vi "Run Tests (Path).vi"(8 "error in (no error)":errorcluster, 10 "Project or Class Path":path, 11 "Execution API In":refnum<class "Execution API.lvclass">) -> (0 "error out":errorcluster, 3 "Execution API Out":refnum<class "Execution API.lvclass">)   [LabVIEW 2020, in "Execution API.lvclass"]
doc: "Run all tests in a project or a test case at the specified path."
uses:
  Execution API.lvclass
  API/LUnit Test Suite/LUnit Test Suite.lvclass
  <vilib>/Utility/error.llb/Error Cluster From Error Code.vi
  <vilib>/ErrorRing/Error Ring.xnode
  Framework/Test Finder/Test Finder.lvclass
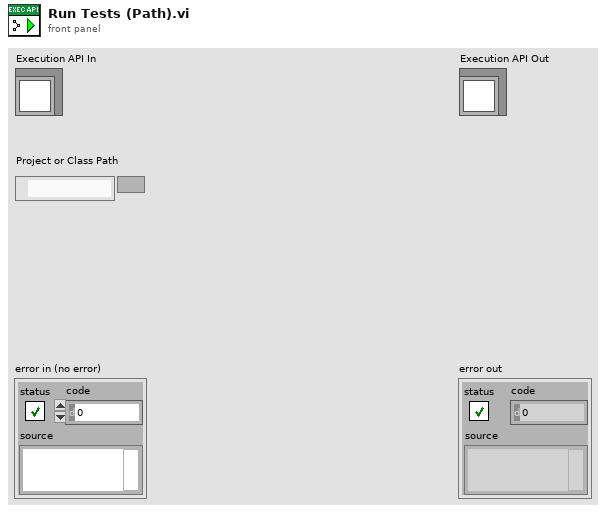
[diagram p1: front panel]
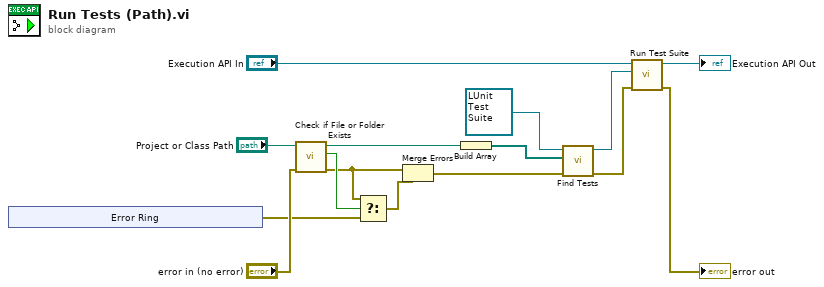
[diagram p0: block diagram]
diagram:
  n1 = xnode "Error Ring"() -> ("error out"=w7:errorcluster)
  n2 = call <vilib>:"Check if File or Folder Exists.vi"("error in (no error)"="error in (no error)", "path"="Project or Class Path") -> ("error out"=w9:errorcluster, "file or folder exists?"=w10:bool, "dup path"=w5:path)  [unwired: 7 in]
  n3 = Select(t=w9, s=w10, f=w7) -> (s? t:f=w8:errorcluster)
  n4 = Merge Errors(w9, w8) -> (w3:errorcluster)
  n5 = Build Array(w5) -> (w4:path[])
  n6 = call "Find Tests.vi"("error in (no error)"=w3, "File Paths"=w4, "LUnit Test Suite"=refnum<class "LUnit Test Suite.lvclass"> refnum) -> ("error out"=w1:errorcluster, "LUnit Test Suite"=w2:refnum<class "LUnit Test Suite.lvclass">)  [unwired: 7 in]
  n7 = call "Run Test Suite.vi"("error in (no error)"=w1, "Test Suite"=w2, "Execution API In"="Execution API In") -> ("error out"=→"error out":errorcluster, "Execution API Out"=→"Execution API Out":refnum<class "Execution API.lvclass">)  [unwired: 7 in]
